vi "CheckForErrorsString.vi"(9 "Parameter Index":dbl, 10 "Allowed values":string[](array[string]), 11 "Parameters":string[](array[string])) -> (2 "Error":errorcluster, 3 "Output":string)   [LabVIEW 2019]
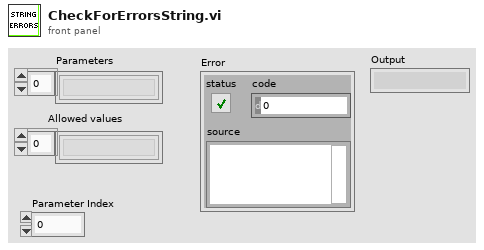
[diagram p1: front panel]
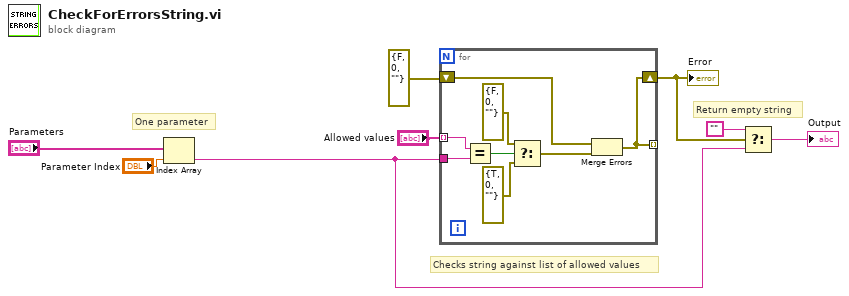
[diagram p0: block diagram]
diagram:
  # "Checks string against list of allowed values"
  # "Return empty string"
  # "One parameter"
  n1 = Index Array(array="Parameters", index="Parameter Index") -> (element=w2:string)
  n2 = for {
    tunnel: "Allowed values" -> [w16] mode=indexing
    tunnel: w2 -> [w15]
    shift-right: [w9] -> w3
    shift-left: errorcluster {"status"=FALSE, "code"=0, "source"=""} ("error constant") -> [w10]
    tunnel: [w9] -> _ mode=indexing
    n3 = Equal?(x=w16, y=w15) -> (x = y?=w14:bool)
    n4 = Select(t=errorcluster {"status"=FALSE, "code"=0, "source"=""} ("error constant"), s=w14, f=errorcluster {"status"=TRUE, "code"=0, "source"=""} ("error constant")) -> (s? t:f=w11:errorcluster)
    n5 = Merge Errors(w10, w11) -> (w9:errorcluster)
  }
  "Error" <- w3
  n6 = Select(t="", s=w3, f=w2) -> (s? t:f=→"Output":string)
